vi "Scale Point 3D (SGL) To Screen.vi"(7 "Screen Dimensions":cluster{"Width":sgl, "Height":sgl}, 11 "Point In":T1) -> (3 "Point Out":T1)   [LabVIEW 2020, in "3D.lvlib"]
uses:
  Vector 3D.ctl
  3D.lvlib
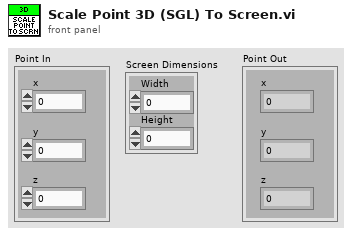
[diagram p1: front panel]
types:
  T1 = typedef "3D.lvlib/Vector 3D.ctl" = cluster{"x":sgl, "y":sgl, "z":sgl}
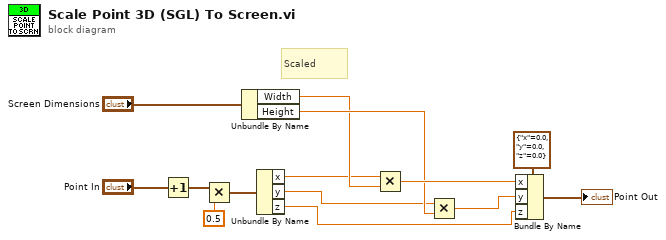
[diagram p0: block diagram]
diagram:
  # "Scaled"
  n1 = Increment(x="Point In") -> (x+1=w2:T1)
  n2 = Multiply(x=w2, y=sgl 0.5 ("x")) -> (x*y=w4:T1)
  n3 = Unbundle By Name("Screen Dimensions") -> ("Width"=w7:sgl, "Height"=w9:sgl)
  n4 = Unbundle By Name(w4) -> ("x"=w6:sgl, "y"=w8:sgl, "z"=w12:sgl)
  n5 = Multiply(x=w6, y=w7) -> (x*y=w10:sgl)
  n6 = Multiply(x=w8, y=w9) -> (x*y=w11:sgl)
  n7 = Bundle By Name(cluster=T1 {"x"=0.0, "y"=0.0, "z"=0.0} ("Vector 3D"), "x"=w10, "y"=w11, "z"=w12) -> (→"Point Out":T1)
